vi "Get Terminal Name with Device Prefix.vi"(8 "error in (no error)":errorcluster, 10 "Local Terminal Name":string, 11 "task/channels in":refnum<k21>) -> (0 "error out":errorcluster, 2 "Terminal Name with Device Prefix":tag, 3 "task out":refnum<k21>)   [LabVIEW 2017]
doc: "This example takes in a DAQmx Task and a terminal and converts this to a terminal which includes the device prefix specified in the DAQmx Physical Channel Control.\n\nFor example: \nDAQmx Task/channels in=Dev1/ai1:2\nTerminal=ai/StartTrigger\nDevice+Terminal=/Dev1/ai/StartTrigger"
uses:
  <resource>/objmgr/daqmx.rc
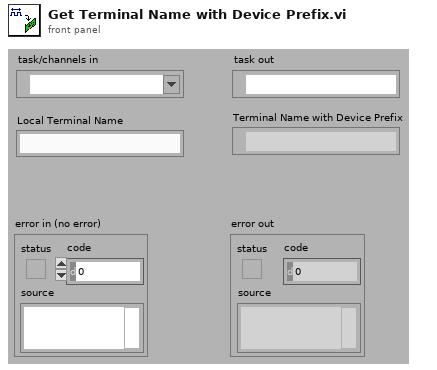
[diagram p1: front panel]
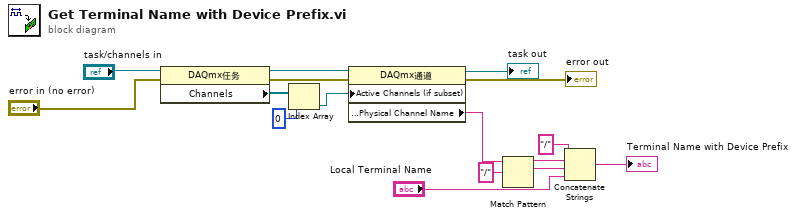
[diagram p0: block diagram]
diagram:
  n1 = property class="DAQmx任务"(reference="task/channels in", error in="error in (no error)") -> (reference out=w1:refnum<k21>, error out=w7:errorcluster, "Channels"=w11:refnum<k21>[])
  n2 = Index Array(array=w11, index=0) -> (element=w9:refnum<k21>)
  n3 = property class="DAQmx通道"(reference=w1, error in=w7, "Active Channels (if subset)"=w9) -> (reference out=→"task out":refnum<k21>, error out=→"error out":errorcluster, "General Properties:Physical Channel Name"=w6:tag)
  n4 = Match Pattern(string=w6, regular expression="/") -> (before substring=w13:string, match substring=w14:string)  [unwired: 1 in, 2 out]
  n5 = Concatenate Strings("/" ("string"), w13, w14, "Local Terminal Name") -> (→"Terminal Name with Device Prefix":string)
